vi "Create.vi"(8 "Error In":errorcluster, 11 "labssh2 Shared Library":path=path "") -> (0 "Error Out":errorcluster, 3 "Sesssion":refnum<class "Session.lvclass">)   [LabVIEW 2017, in "LabSSH2.lvlib" / "Session.lvclass"]
uses:
  Session.lvclass
  Session.lvclass/Session.ctl
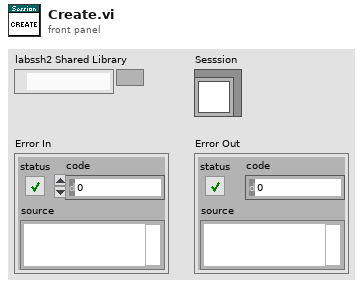
[diagram p1: front panel]
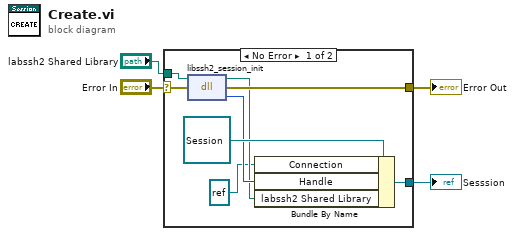
[diagram p0: block diagram]
diagram:
  n1 = case shown="No Error" "Error In" {
    selector: "Error In" -> [w10 w13]
    tunnel: [w11 _] -> w3
    tunnel: "labssh2 Shared Library" -> [w9 _]
    tunnel: [w8 w13] -> w1
    frame No Error {
      n2 = dll-call lib="D:/Users/cfield/Code/Field R&D Services/SSH/LabSSH2/LabVIEW/trunk/src/LabSSH2/Private/labssh2.*" fn="libssh2_session_init"(path in=w9, error in=w10) -> (path out=w6:path, error out=w8:errorcluster, "SESSION"=w7:u64)  [unwired: 1 in]
      n3 = Bundle By Name(cluster=refnum<class "Session.lvclass"> refnum ("LabSSH2.lvlib:Session.lvclass"), "Connection"=refnum<k5> refnum, "Handle"=w7, "labssh2 Shared Library"=w6) -> (w11:refnum<class "Session.lvclass">)
    }
    frame Error {
    }
  }
  "Sesssion" <- w3
  "Error Out" <- w1
